vi "resonancia.vi"() -> ()   [LabVIEW 2010]
uses:
  <vilib>/sound2/lvsound2.llb/Sound Data Format.ctl
  <vilib>/sound2/lvsound2.llb/Sampling Mode.ctl
  <vilib>/sound2/lvsound2.llb/Sound Input Read (DBL).vi
  <vilib>/sound2/lvsound2.llb/Sound Output Write (DBL Single).vi
  <vilib>/measure/madcrms.llb/Basic Averaged DC-RMS for 1 Chan.vi
  <vilib>/measure/matone.llb/Extract Single Tone Information 1 Chan.vi
  <vilib>/measure/NI_MAPro.lvlib
panel:
  in  "Grabar?":bool
  out "tiempo":dbl
  in  "number of samples/ch":i32=20000
  out "x/y":dbl
  out "Frecuencia":i32
  in  "Sound Format":T1={"sample rate (S/s)"=44100.0, "number of channels"=2, "bits per sample"=16}
  in  "Input Device ID":u32
  in  "Output Device ID":u32
  in  "stop":bool
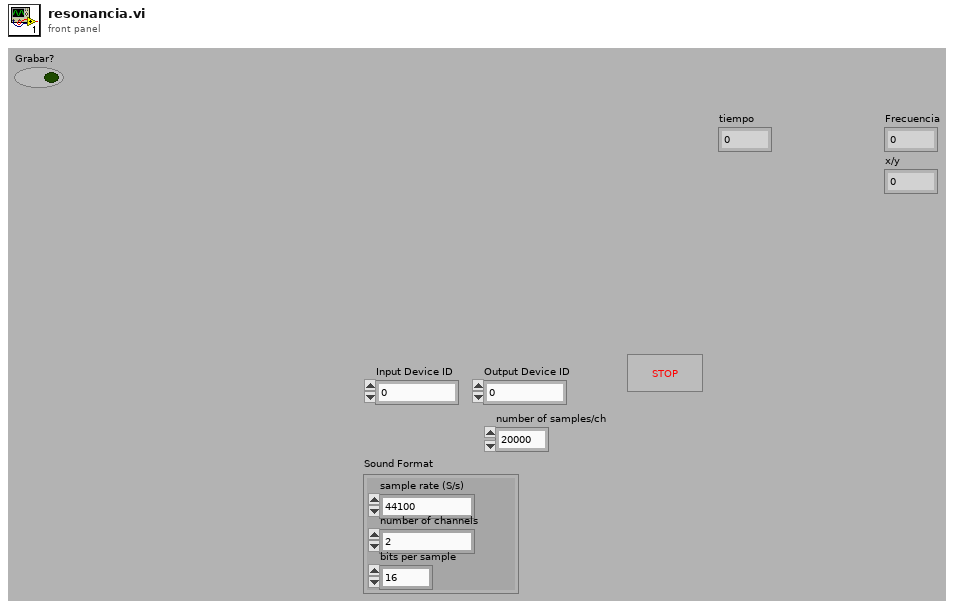
[diagram p1: front panel]
types:
  T1 = typedef "Sound Data Format.ctl" = cluster{"sample rate (S/s)":dbl, "number of channels":i32, "bits per sample":i32}
  T2 = enum32{"existing file", "new file", "new or existing file", "existing dir", "new dir", "new or existing dir", "existing file (use LLBs)", "new file (use LLBs)", "new or existing file (use LLBs)", "new or existing file or directory (use LLBs)"}
  T3 = enum16{"open", "replace", "create", "open or create", "replace or create", "replace or create with confirmation"}
  T4 = typedef "Sampling Mode.ctl" = i32
  T5 = typedef "Sound Output Task ID.ctl" = u32
  T6 = typedef "Sound Input Task ID.ctl" = u32
  T7 = cluster{"approx freq. (optional)":dbl, "search (+/- % of Fsampl.)":dbl}
  T8 = enum32{"none", "input signal", "detected signal", "residual signal"}
  T9 = cluster{"averaging mode":enum16{"No averaging", "Vector averaging", "RMS averaging", "Peak hold"}, "weighting mode":enum16{"Linear", "Exponential"}, "number of averages":u32}
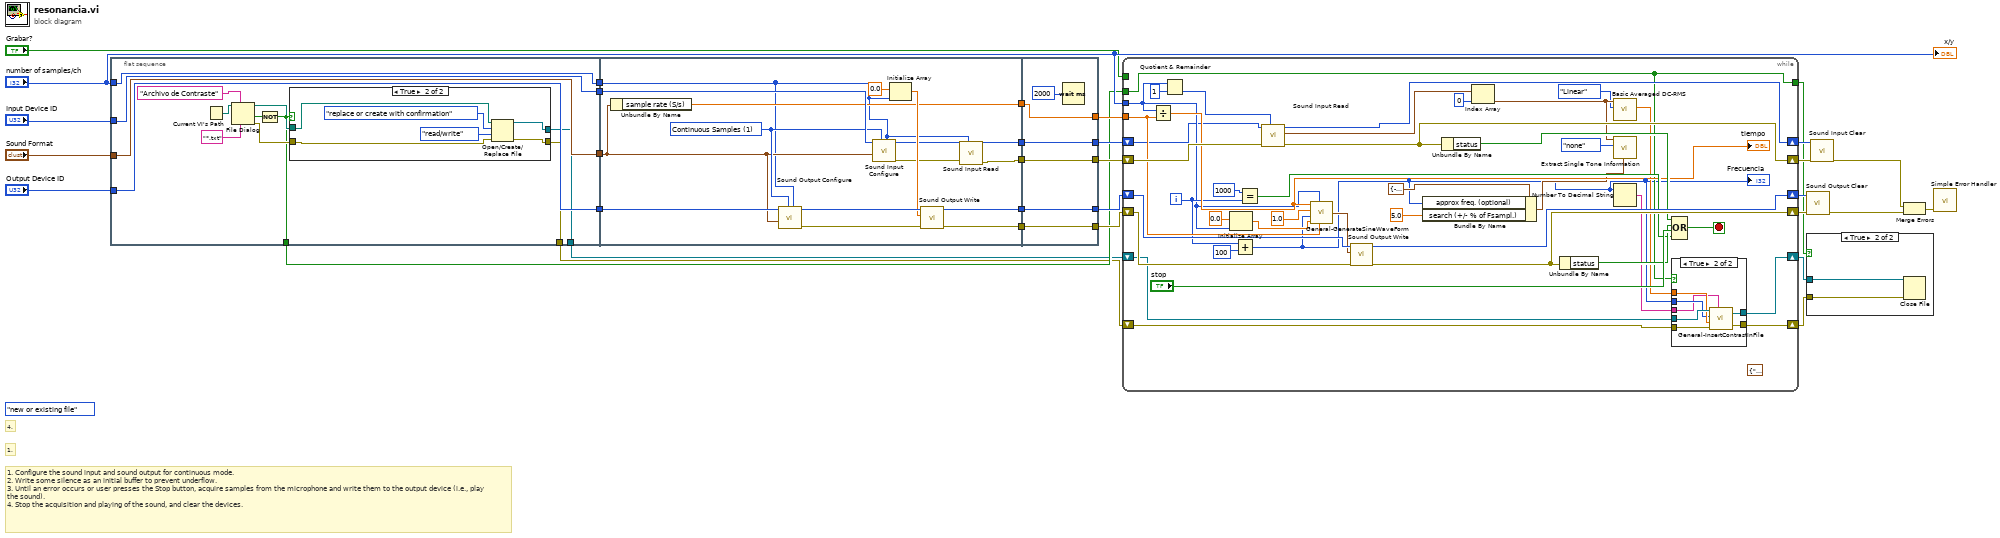
[diagram p0: block diagram]
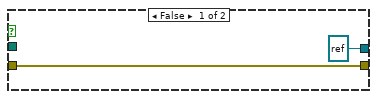
[diagram p2: hidden frame]
diagram:
  (unwired) T2."new or existing file" ("select mode (2)")
  # "4."
  # "1."
  # "1. Configure the sound input and sound output for continuous mode.\n2. Write some silence as an initial buffer to prevent underflow.\n3. Until an error occurs or user presses the Stop button, acquire samples from the microphone and write them to the output device (i.e., play the sound).\n4. Stop the acquisition and playing of the sound, and clear the devices."
  n1 = flat-sequence {
    tunnel: "number of samples/ch" -> [w42]
    tunnel: "Sound Format" -> [w43]
    tunnel: "Input Device ID" -> [w44]
    tunnel: "Output Device ID" -> [w45]
    tunnel: [w45] -> w13
    tunnel: [w44] -> w12
    tunnel: [w43] -> w11
    tunnel: [w42] -> w10
    tunnel: [w35] -> w9
    tunnel: [w34] -> w8
    tunnel: [w33] -> w7
    tunnel: w13 -> [w69]
    tunnel: w12 -> [w68]
    tunnel: w11 -> [w60]
    tunnel: w10 -> [w54]
    tunnel: [w56] -> w5
    tunnel: [w64] -> w4
    tunnel: [w63] -> w3
    tunnel: [w59] -> w2
    tunnel: [w55] -> w1
    tunnel: [w71] -> w18
    tunnel: [w72] -> w21
    tunnel: [w73] -> w22
    tunnel: [w74] -> w23
    tunnel: [w75] -> w24
    tunnel: w5 -> [w75]
    tunnel: w4 -> [w73]
    tunnel: w3 -> [w72]
    tunnel: w2 -> [w71]
    tunnel: w1 -> [w74]
    frame #0 {
      n2 = Current VI's Path() -> (path=w38:path)
      n3 = File Dialog(6:"*.txt" ("pattern"), 7:"Archivo de Contraste" ("prompt"), 11:w38) -> (0:w37:errorcluster, 1:w39:bool, 3:w36:path)  [unwired: 1 in, 4 out]
      n4 = Not(x=w39) -> (.not. x?=w35:bool)
      n5 = case shown="True" w35 {
        tunnel: w37 -> [w47 w53]
        tunnel: w36 -> [_ w52]
        tunnel: [refnum<file> refnum ("refnum out") w51] -> w34
        tunnel: [w47 w50] -> w33
        frame False {
        }
        frame True {
          n6 = Open/Create/Replace File(file path (use dialog)=w52, error in=w53, operation (0:open)=T3."replace or create with confirmation", access (0:read/write)=enum16{"read/write", "read-only", "write-only"}."read/write") -> (refnum out=w51:refnum<file>, error out=w50:errorcluster)  [unwired: 2 in, 1 out]
        }
      }
    }
    frame #1 {
      w67 = T4 1 items=["Finite Samples", "Continuous Samples"] ("sample mode")
      n7 = Unbundle By Name(w60) -> ("sample rate (S/s)"=w59:dbl)
      n8 = call <vilib>:"Sound Output Configure.vi"("number of samples/ch"=w54, "sample mode"=w67, "sound format"=w60, "device ID"=w69) -> ("error out"=w65:errorcluster, "task ID"=w66:T5)  [unwired: 6 in]
      n9 = call <vilib>:"Sound Input Configure.vi"("number of samples/ch"=w54, "sample mode"=w67, "sound format"=w60, "device ID"=w68) -> ("error out"=w57:errorcluster, "task ID"=w58:T6)  [unwired: 6 in]
      n10 = Initialize Array(0.0 ("element"), w54) -> (w61:dbl[])
      n11 = call-poly <vilib>:"Sound Output Write.vi"("error in (no error)"=w65, "data"=w61, "task ID"=w66) -> ("error out"=w64:errorcluster, "task ID out"=w63:T5)  [unwired: 7 in]
      n12 = call-poly <vilib>:"Sound Input Read.vi"("number of samples/ch"=w54, "error in (no error)"=w57, "task ID"=w58) -> ("error out"=w56:errorcluster, "task ID out"=w55:T6)  [unwired: 6 in, 1 out]
    }
    frame #2 {
      n13 = Wait (ms)(milliseconds to wait=u32 2000) -> ()  [unwired: 1 out]
    }
  }
  n14 = while {
    shift-right: [w110] -> w31
    shift-left: w22 -> [w112]
    shift-right: [w111] -> w32
    shift-left: w24 -> [w116]
    shift-right: [w114] -> w30
    shift-left: w21 -> [w115]
    shift-right: [w113] -> w27
    shift-left: w23 -> [w82]
    tunnel: w18 -> [w99]
    tunnel: "number of samples/ch" -> [w86]
    tunnel: w9 -> [w88]
    tunnel: [w88] -> w14
    shift-right: [w89] -> w15
    shift-left: w8 -> [w94]
    shift-right: [w90] -> w16
    shift-left: w7 -> [w93]
    tunnel: "Grabar?" -> [_]
    i -> [w96]
    stop <- w106 stop-if-true
    (unwired) T9 {"averaging mode"=enum."RMS averaging", "weighting mode"=enum."Linear", "number of averages"=10} ("averaging parameters")
    n15 = Divide(x=w86, y=w99) -> (x/y=w98:dbl)
    "tiempo" <- w98
    n16 = Quotient & Remainder(x=w86, y=u32 1 ("x")) -> (floor(x/y)=w81:u32)  [unwired: 1 out]
    n17 = Initialize Array(0.0 ("element"), w86) -> (w104:dbl[])
    n18 = Add(x=w96, y=100) -> (x+y=w76:i32)
    "Frecuencia" <- w76
    n19 = Equal?(x=1000, y=w96) -> (x = y?=w102:bool)
    n20 = call-poly <vilib>:"Sound Input Read.vi"("number of samples/ch"=w81, "error in (no error)"=w116, "task ID"=w82) -> ("error out"=w111:errorcluster, "data"=w80:waveform(dbl)[], "task ID out"=w113:T6)  [unwired: 6 in]
    n21 = call "General-GenerateSineWaveForm.vi"("tiempo (s)"=w98, "#samples"=w86, "Amplitud"=1.0, "frecuencia"=w76, "Fs (S/s)"=w99, "df"=w104) -> ("Waveform"=w100:waveform(dbl))  [unwired: 2 in]
    n22 = call-poly <vilib>:"Sound Output Write.vi"("error in (no error)"=w112, "data"=w100, "task ID"=w115) -> ("error out"=w110:errorcluster, "task ID out"=w114:T5)  [unwired: 7 in]
    n23 = Bundle By Name(cluster=T7 {"approx freq. (optional)"=-1.0, "search (+/- % of Fsampl.)"=5.0} ("advanced search"), "approx freq. (optional)"=w76, "search (+/- % of Fsampl.)"=5.0) -> (w91:T7)
    n24 = Unbundle By Name(w111) -> ("status"=w107:bool)
    n25 = Index Array(array=w80, index=0) -> (element=w79:waveform(dbl))
    n26 = Unbundle By Name(w110) -> ("status"=w108:bool)
    n27 = call-poly <vilib>:"Basic Averaged DC-RMS.vi"("averaging type"=enum16{"Linear", "Exponential"}."Linear", "signal in"=w79) -> ("RMS value"=w77:dbl)  [unwired: 6 in, 3 out]
    n28 = call-poly <vilib>:"Extract Single Tone Information.vi"("advanced search"=w91, "export mode"=T8."none", "time signal in"=w79) -> ()  [unwired: 3 in, 6 out]
    n29 = Number To Decimal String(number=w76) -> (decimal integer string=w84:string)  [unwired: 1 in]
    n30 = Compound Arithmetic op=OR(w107, w108, "stop", w102) -> (w106:bool)
    n31 = case shown="True" w88 {
      tunnel: w94 -> [w118 w125]
      tunnel: w93 -> [w117 w124]
      tunnel: w77 -> [_ w123]
      tunnel: w76 -> [_ w122]
      tunnel: [w117 w121] -> w90
      tunnel: [w118 w120] -> w89
      tunnel: w84 -> [_ w119]
      frame False {
      }
      frame True {
        n32 = call "General-InsertContrastInFile.vi"("refnum IN"=w125, "tiempo (ms)"=w122, "contraste"=w123, "error IN"=w124, "Status"=w119) -> ("refnum OUT"=w120:refnum<file>, "error OUT"=w121:errorcluster)
      }
    }
  }
  n33 = call <vilib>:"Sound Output Clear.vi"("error in (no error)"=w31, "task ID"=w30) -> ("error out"=w26:errorcluster)  [unwired: 9 in]
  n34 = case shown="True" w14 {
    tunnel: w16 -> [_ w127]
    tunnel: w15 -> [_ w126]
    frame False {
    }
    frame True {
      n35 = Close File(refnum=w126, error in=w127) -> ()  [unwired: 2 out]
    }
  }
  n36 = call <vilib>:"Sound Input Clear.vi"("error in (no error)"=w32, "task ID"=w27) -> ("error out"=w25:errorcluster)  [unwired: 9 in]
  n37 = Merge Errors(w25, w26) -> (w20:errorcluster)
  n38 = call <vilib>:"Simple Error Handler.vi"("error in (no error)"=w20) -> ()  [unwired: 4 in, 5 out]
  "x/y" <- "number of samples/ch"
